vi "Write Memory.vi"(9 "Data to write (HEX, max 16 bytes)":string, 10 "Page Address":i32 format="%x", 11 "PN532 COM Port":refnum<visa-resource-name>) -> (0 "Error Out":errorcluster, 2 "Succesful?":bool, 3 "PN532 COM Port Out":refnum<visa-resource-name>)   [LabVIEW 2012, in "NFC Driver.lvlib"]
doc: "This VI writes to the NTAG's memory the data contained in \"Data to write (max 16 bytes)\" to the page specified in \"Page\".\n\nThe maximum size of the data to write is 16 bytes or 4 characters. Any data larger than 16 bytes will be truncated."
uses:
  NFC Driver.lvlib
panel:
  out "substring":string
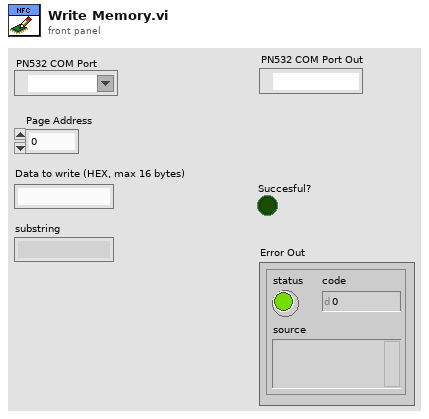
[diagram p1: front panel]
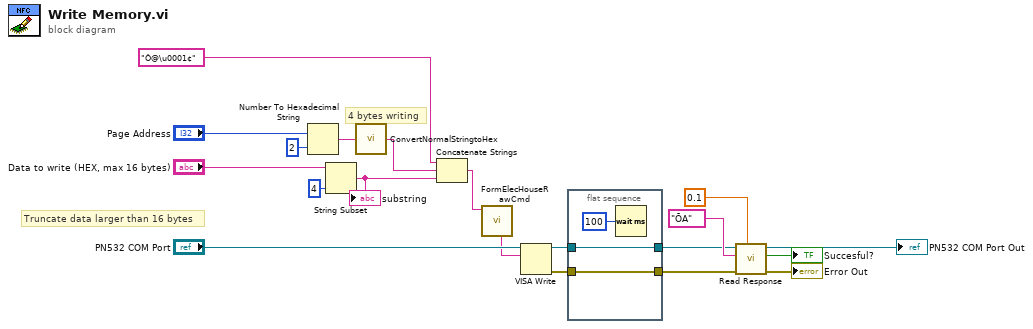
[diagram p0: block diagram]
diagram:
  # "Truncate data larger than 16 bytes"
  # "4 bytes writing"
  n1 = Number To Hexadecimal String(1:i16 2 ("width (-)"), 2:"Page Address") -> (0:w4:string)
  n2 = String Subset(string="Data to write (HEX, max 16 bytes)", length (rest)=4 ("length (rest)")) -> (substring=w10:string)  [unwired: 1 in]
  "substring" <- w10
  n3 = call "ConvertNormalStringtoHex.vi"("Normal String"=w4) -> ("Hex String"=w3:string)
  n4 = Concatenate Strings("Ô@\u0001¢" ("string"), w3, w10) -> (w14:string)
  n5 = call "FormElecHouseRawCmd.vi"("Command"=w14) -> ("concatenated Cmd"=w19:string)  [unwired: 10 in]
  n6 = VISA Write(VISA resource name="PN532 COM Port", write buffer=w19) -> (VISA resource name out=w9:refnum<visa-resource-name>, error out=w7:errorcluster)  [unwired: 1 in, 1 out]
  n7 = flat-sequence {
    tunnel: w9 -> [w22]
    tunnel: [w22] -> w8
    tunnel: w7 -> [w21]
    tunnel: [w21] -> w6
    frame #0 {
      n8 = Wait (ms)(milliseconds to wait=u32 100) -> ()  [unwired: 1 out]
    }
  }
  n9 = call "Read Response.vi"("Timeout (s)"=0.1, "error in (no error)"=w6, "regular expression"="ÕA", "PN532 COM Port"=w8) -> ("error out"=→"Error Out":errorcluster, "Found?"=→"Succesful?":bool, "PN532 COM Port Out"=→"PN532 COM Port Out":refnum<visa-resource-name>)  [unwired: 4 in, 1 out]
